vi "PullBack.vi"(6 "Output":dbl=1.0 format="%#_13g", 8 "error in (no error)":errorcluster, 9 "dog shifter timeout (s)":i32, 10 "winch timeout (s)":i32) -> (0 "error out":errorcluster)   [LabVIEW 2013]
uses:
  <vilib>/Rock Robotics/WPI/CAN/Jaguar/SubVIs/WPI_CANJaguar_StatusSelect.ctl
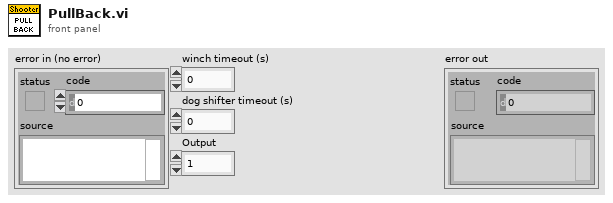
[diagram p1: front panel]
types:
  T1 = typedef "WPI_CANJaguar_StatusSelect.ctl" = enum16{"Output Percent VBus", "Output Voltage", "Bus Voltage", "Current", "Temperature", "Position", "Speed", "Limit Switches", "Faults", "Fault Counters", "Power Cycle"}
  T2 = typedef "WPI_MotorControlDeviceRef.ctl" = cluster{"DeviceStatus":errorcluster, "Type":enum16{"PWM", "CAN"}, "PWM":cluster{"Digital Module":T3, "PWM Channel":T4, "DeadBand":T5}, "CAN":cluster{"Device Number":u8, "Control Mode":T6, "Semaphore":T7, "Max Vout":dbl}, "Invert":bool, "TransformRef":T8, "InvTransformRef":T8}
  T3 = typedef "FPGA_TypedefDigitalModule.ctl" = enum16{"Digital Module 1", "Digital Module 2"}
  T4 = typedef "FPGA_DIOPWMChannel.ctl" = enum8{"PWM 1", "PWM 2", "PWM 3", "PWM 4", "PWM 5", "PWM 6", "PWM 7", "PWM 8", "PWM 9", "PWM 10", "Invalid"}
  T5 = typedef "WPI_PWMDeadband.ctl" = cluster{"Name":string, "maxPositivePwm":i32, "minPositivePwm":i32, "centerPwm":i32, "maxNegativePwm":i32, "minNegativePwm":i32, "angularRange":u16}
  T6 = typedef "WPI_CANJaguar_ControlMode.ctl" = enum8{"Percent VBus", "Current", "Speed", "Position", "Voltage"}
  T7 = typedef "Semaphore RefNum" = refnum<k1>
  T8 = typedef "WPI_PWMTransform_ConPane.ctl" = refnum<vi>
  T9 = typedef "WPI_CANJaguar_Status.ctl" = cluster{"Output Percent VBus":dbl, "Output Voltage":dbl, "Bus Voltage":dbl, "Current":dbl, "Temperature":dbl, "Position":dbl, "Speed":dbl, "Limits":cluster{"Forward Limit":bool, "Reverse Limit":bool, "Forward Soft Limit":bool, "Reverse Soft Limit":bool, "Sticky Forward Limit":bool, "Sticky Reverse Limit":bool, "Sticky Forward Soft Limit":bool, "Sticky Reverse Soft Limit":bool}, "Faults":cluster{"Current Fault":bool, "Temperature Fault":bool, "Bus Voltage Fault":bool, "Gate Driver Fault":bool, "Comm Fault":bool}, "Fault Counters":cluster{"Current Faults":u8, "Temperature Faults":u8, "Bus Voltage Faults":u8, "Gate Driver Faults":u8, "Comm Faults":u8, "CAN Status":u8, "CAN RX Errors":u8, "CAN TX Errors":u8}, "Power Cycle":bool}
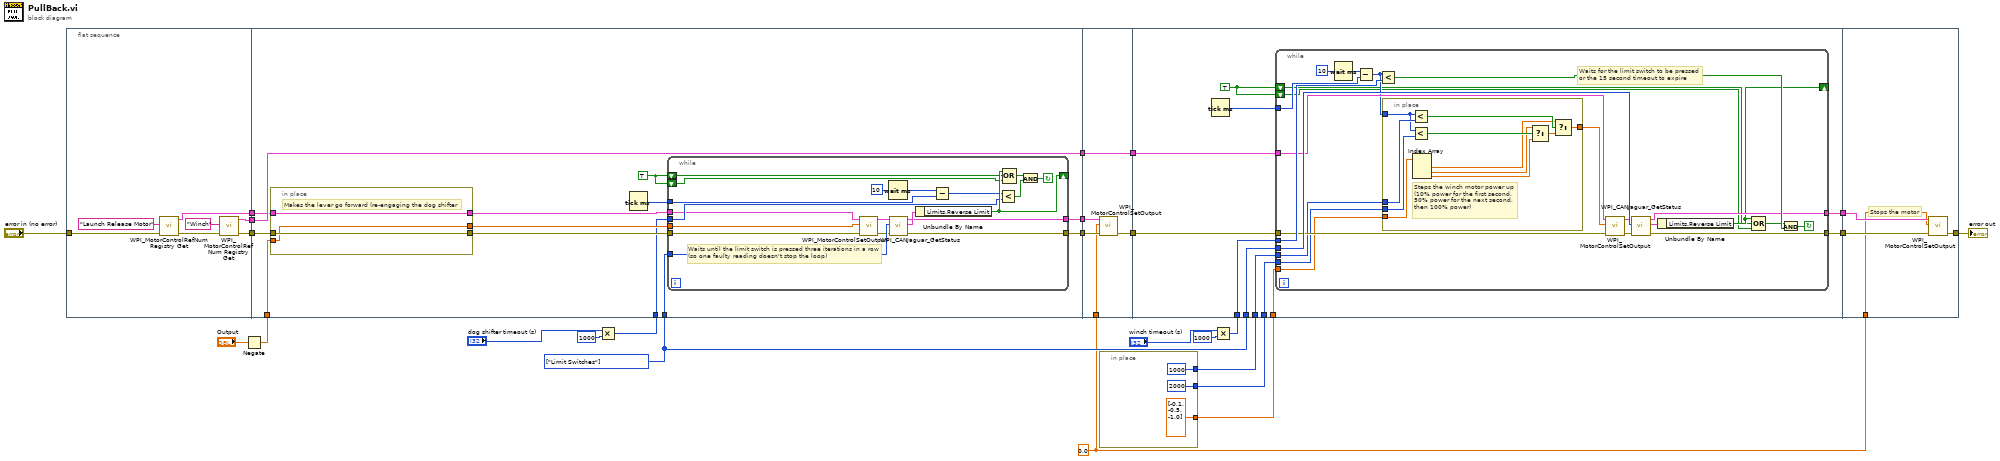
[diagram p0: block diagram]
diagram:
  w6 = 0.0 ("Output")
  w11 = T1[] [enum."Limit Switches"] items=["Output Percent VBus", "Output Voltage", "Bus Voltage", "Current", "Temperature", "Position", "Speed", "Limit Switches", "Faults", "Fault Counters", "Power Cycle"] ("Status Select")
  n1 = flat-sequence {
    tunnel: "error in (no error)" -> [w28]
    tunnel: [w30] -> w15
    tunnel: [w31] -> w14
    tunnel: [w26] -> w13
    tunnel: w15 -> [w43]
    tunnel: w14 -> [w45]
    tunnel: [w45] -> w9
    tunnel: w13 -> [w44]
    tunnel: w1 -> [w42]
    tunnel: w11 -> [w37]
    tunnel: [w33] -> w7
    tunnel: w5 -> [w35]
    tunnel: [w34] -> w2
    tunnel: [w71] -> w10
    tunnel: w9 -> [w73]
    tunnel: [w73] -> w8
    tunnel: w7 -> [w70]
    tunnel: w6 -> [w69]
    tunnel: w2 -> [w72]
    tunnel: w10 -> [w78]
    tunnel: [w81] -> w24
    tunnel: [w80] -> w23
    tunnel: w11 -> [w84]
    tunnel: w8 -> [w79]
    tunnel: w19 -> [w82]
    tunnel: w18 -> [w77]
    tunnel: w17 -> [w76]
    tunnel: w16 -> [w75]
    tunnel: w24 -> [w122]
    tunnel: w23 -> [w121]
    tunnel: [w120] -> w22
    tunnel: w6 -> [w119]
    frame #0 {
      n2 = call <vilib>:"WPI_MotorControlRefNum Registry Get.vi"("error in (no error)"=w28, "refnum name"="Launch Release Motor") -> ("error out"=w27:errorcluster, "MotorControlDevRef"=w26:T2)  [unwired: 8 in]
      n3 = call <vilib>:"WPI_MotorControlRefNum Registry Get.vi"("error in (no error)"=w27, "refnum name"="Winch") -> ("error out"=w30:errorcluster, "MotorControlDevRef"=w31:T2)  [unwired: 8 in]
    }
    frame #1 {
      w41 = TRUE
      n4 = in-place {
        in-place-border: w44 -> [w67]
        in-place-border: w43 -> [w68]
        in-place-border: w42 -> [w66]
        in-place-border: [w68] -> w39
        in-place-border: [w67] -> w40
        in-place-border: [w66] -> w38
        # "Makes the lever go forward (re-engaging the dog shifter"
      }
      n5 = Tick Count (ms)() -> (millisecond timer value=w36:u32)
      n6 = while {
        tunnel: w37 -> [w63]
        tunnel: [w62] -> w34
        shift-right: [w61] -> _
        shift-left: w41 -> [w60]
        shift-left: w41 -> [w59]
        tunnel: [w64] -> w33
        tunnel: w36 -> [w54]
        tunnel: w35 -> [w51]
        tunnel: w39 -> [w49]
        tunnel: w40 -> [w48]
        tunnel: w38 -> [w47]
        stop <- w53 continue-if-true
        # "Waits until the limit switch is pressed three iterations in a row\n(so one faulty reading doesn't stop the loop)"
        n7 = call <vilib>:"WPI_MotorControlSetOutput.vi"("error in (no error)"=w49, "Output"=w47, "MotorControlDevRef"=w48) -> ("error out"=w50:errorcluster, "MotorControlDevRef"=w46:T2)  [unwired: 6 in, 1 out]
        n8 = Wait (ms)(milliseconds to wait=u32 10) -> (millisecond timer value=w56:u32)
        n9 = call <vilib>:"WPI_CANJaguar_GetStatus.vi"("error in (no error)"=w50, "Status Select"=w63, "CAN Jaguar Ref"=w46) -> ("error out"=w62:errorcluster, "Status"=w65:T9, "CAN Jaguar Ref Out"=w64:T2)  [unwired: 6 in]
        n10 = Unbundle By Name(w65) -> ("Limits.Reverse Limit"=w61:bool)
        n11 = Subtract(x=w56, y=w54) -> (x-y=w57:u32)
        n12 = Less?(x=w57, y=w51) -> (x < y?=w52:bool)
        n13 = Compound Arithmetic op=OR(w61, w60, w59) -> (w58:bool)
        n14 = And(x=w58, y=w52) -> (x .and. y?=w53:bool)
      }
    }
    frame #2 {
      n15 = call <vilib>:"WPI_MotorControlSetOutput.vi"("error in (no error)"=w72, "Output"=w69, "MotorControlDevRef"=w70) -> ("error out"=w71:errorcluster)  [unwired: 6 in, 2 out]
    }
    frame #3 {
      w74 = TRUE ("Reverse Limit")
      n16 = Tick Count (ms)() -> (millisecond timer value=w83:u32)
      n17 = while {
        tunnel: w84 -> [w105]
        tunnel: w83 -> [w102]
        tunnel: w82 -> [w101]
        tunnel: w78 -> [w94]
        tunnel: [w99] -> w81
        tunnel: w79 -> [w95]
        tunnel: [w98] -> w80
        tunnel: w77 -> [w93]
        tunnel: w76 -> [w91]
        tunnel: w75 -> [w89]
        shift-right: [w88] -> _
        shift-left: w74 -> [w87]
        shift-left: w74 -> [w86]
        stop <- w104 continue-if-true
        # "Waits for the limit switch to be pressed\nor the 15 second timeout to expire"
        n18 = Wait (ms)(milliseconds to wait=u32 10) -> (millisecond timer value=w100:u32)
        n19 = Subtract(x=w100, y=w102) -> (x-y=w92:u32)
        n20 = Less?(x=w92, y=w101) -> (x < y?=w103:bool)
        n21 = in-place {
          in-place-border: w93 -> [w118]
          in-place-border: w92 -> [w116]
          in-place-border: w91 -> [w115]
          in-place-border: [w113] -> w90
          in-place-border: w89 -> [w111]
          # "Steps the winch motor power up\n(10% power for the first second,\n50% power for the next second,\nthen 100% power)"
          n22 = Less?(x=w116, y=w118) -> (x < y?=w117:bool)
          n23 = Less?(x=w116, y=w115) -> (x < y?=w112:bool)
          n24 = Index Array(array=w111) -> (element #1=w110:dbl, element #2=w109:dbl, element #3=w108:dbl)  [unwired: 3 in]
          n25 = Select(t=w109, s=w112, f=w108) -> (s? t:f=w114:dbl)
          n26 = Select(t=w110, s=w117, f=w114) -> (s? t:f=w113:dbl)
        }
        n27 = call <vilib>:"WPI_MotorControlSetOutput.vi"("error in (no error)"=w94, "Output"=w90, "MotorControlDevRef"=w95) -> ("error out"=w97:errorcluster, "MotorControlDevRef"=w96:T2)  [unwired: 6 in, 1 out]
        n28 = call <vilib>:"WPI_CANJaguar_GetStatus.vi"("error in (no error)"=w97, "Status Select"=w105, "CAN Jaguar Ref"=w96) -> ("error out"=w99:errorcluster, "Status"=w107:T9, "CAN Jaguar Ref Out"=w98:T2)  [unwired: 6 in]
        n29 = Unbundle By Name(w107) -> ("Limits.Reverse Limit"=w88:bool)
        n30 = Compound Arithmetic op=OR(w88, w87, w86) -> (w85:bool)
        n31 = And(x=w85, y=w103) -> (x .and. y?=w104:bool)
      }
    }
    frame #4 {
      # "Stops the motor"
      n32 = call <vilib>:"WPI_MotorControlSetOutput.vi"("error in (no error)"=w122, "Output"=w119, "MotorControlDevRef"=w121) -> ("error out"=w120:errorcluster)  [unwired: 6 in, 2 out]
    }
  }
  n33 = Negate(x="Output") -> (-x=w1:dbl)
  n34 = Multiply(x="dog shifter timeout (s)", y=1000) -> (x*y=w5:i32)
  n35 = in-place {
    in-place-border: [u32 1000 ("y")] -> w18
    in-place-border: [u32 2000 ("y")] -> w17
    in-place-border: [dbl[] [-0.1, -0.5, -1.0]] -> w16
  }
  n36 = Multiply(x="winch timeout (s)", y=1000) -> (x*y=w19:i32)
  "error out" <- w22
